vi "Initialization VI.vi"(8 "error in (no error)":errorcluster, 10 "Custom XML":string, 11 "Device Item Ref in":T1 format="%.0x") -> (0 "error out":errorcluster, 3 "Device Item Ref out":T1 format="%.0x")   [LabVIEW 2019, in "SLSC-12201 DIO System Explorer.lvlib"]
uses:
  SLSC-12201 DIO System Explorer.lvlib
  <vilib>/NI VeriStand/Custom Device API/Custom Device Item Ref.ctl
  Shared/Constants.vi
  <vilib>/NI VeriStand/Custom Device API/Set Item Property (String).vi
  <vilib>/NI VeriStand/Custom Device API/Set Item Property (U32).vi
  <vilib>/NI VeriStand/Custom Device API/Set Item Property (I32).vi
  <vilib>/NI VeriStand/Custom Device API/Get Item Property (Boolean).vi
  <vilib>/NI VeriStand/Custom Device API/Custom Device API.lvlib
  Shared/SLSC-12201 DIO Shared.lvlib
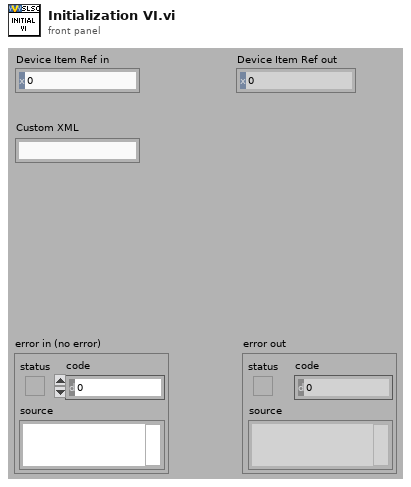
[diagram p1: front panel]
types:
  T1 = typedef "Custom Device API.lvlib/Custom Device Item Ref.ctl" = u64
  T2 = typedef "Custom Device API.lvlib/Custom Device Channel.ctl" = cluster{"Type":T3, "Units":string, "Default Value":dbl, "Faultable":bool, "Scalable":bool}
  T3 = typedef "Custom Device API.lvlib/Custom Device Channel Type.ctl" = enum16{"Input", "Output"}
  T4 = cluster{"Channel Name":string, "SLSC Name":string, "Channel":T2}[]
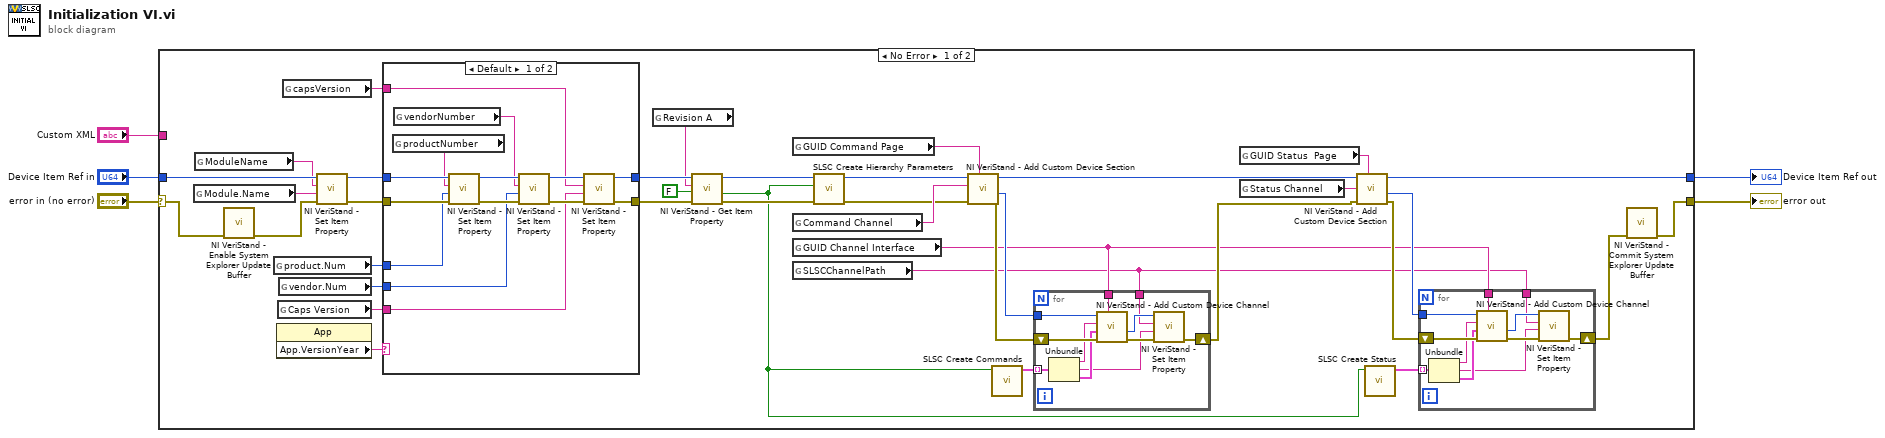
[diagram p0: block diagram]
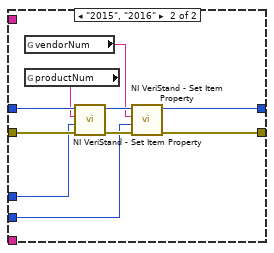
[diagram p2: hidden frame]
diagram:
  n1 = case shown="No Error" "error in (no error)" {
    selector: "error in (no error)" -> [w16 w91]
    tunnel: [w13 w91] -> w5
    tunnel: [w24 w90] -> w3
    tunnel: "Device Item Ref in" -> [w41 w90]
    tunnel: "Custom XML" -> [_ _]
    frame No Error {
      n2 = global read "Constants.vi" "Module.Name"() -> (w39:string)
      n3 = global read "Constants.vi" "ModuleName"() -> (w40:string)
      n4 = call <vilib>:"NI VeriStand - Enable System Explorer Update Buffer.vi"("error in (no error)"=w16) -> ("error out"=w15:errorcluster)  [unwired: 10 in]
      n5 = global read "Constants.vi" "product.Num"() -> (w38:i32)
      n6 = property class="App"() -> ("App.VersionYear"=w19:string)  [unwired: 2 in, 2 out]
      n7 = global read "Constants.vi" "Caps Version"() -> (w17:string)
      n8 = global read "Constants.vi" "vendor.Num"() -> (w37:i32)
      n9 = global read "Constants.vi" "capsVersion"() -> (w18:string)
      n10 = call-poly <vilib>:"NI VeriStand - Set Item Property.vi"("error in (no error)"=w15, "Value"=w39, "Property Name"=w40, "Item Ref in"=w41) -> ("error out"=w42:errorcluster, "Item Ref out"=w43:T1)  [unwired: 5 in, 1 out]
      n11 = case shown="Default" w19 {
        tunnel: w43 -> [w57 w67]
        tunnel: w42 -> [w55 w65]
        tunnel: [w50 w63] -> w12
        tunnel: [w48 w62] -> w11
        tunnel: w38 -> [w53 w61]
        tunnel: w37 -> [w52 w60]
        tunnel: w18 -> [w47 _]
        tunnel: w17 -> [w46 _]
        frame Default {
          n12 = global read "Constants.vi" "productNumber"() -> (w45:string)
          n13 = global read "Constants.vi" "vendorNumber"() -> (w44:string)
          n14 = call-poly <vilib>:"NI VeriStand - Set Item Property.vi"("error in (no error)"=w55, "Value"=w53, "Property Name"=w45, "Item Ref in"=w57) -> ("error out"=w54:errorcluster, "Item Ref out"=w56:T1)  [unwired: 5 in, 1 out]
          n15 = call-poly <vilib>:"NI VeriStand - Set Item Property.vi"("error in (no error)"=w54, "Value"=w52, "Property Name"=w44, "Item Ref in"=w56) -> ("error out"=w49:errorcluster, "Item Ref out"=w51:T1)  [unwired: 5 in, 1 out]
          n16 = call-poly <vilib>:"NI VeriStand - Set Item Property.vi"("error in (no error)"=w49, "Value"=w46, "Property Name"=w47, "Item Ref in"=w51) -> ("error out"=w48:errorcluster, "Item Ref out"=w50:T1)  [unwired: 5 in, 1 out]
        }
        frame "2015", "2016" {
          n17 = global read "Constants.vi" "vendorNum"() -> (w58:string)
          n18 = global read "Constants.vi" "productNum"() -> (w59:string)
          n19 = call-poly <vilib>:"NI VeriStand - Set Item Property.vi"("error in (no error)"=w65, "Value"=w61, "Property Name"=w59, "Item Ref in"=w67) -> ("error out"=w64:errorcluster, "Item Ref out"=w66:T1)  [unwired: 5 in, 1 out]
          n20 = call-poly <vilib>:"NI VeriStand - Set Item Property.vi"("error in (no error)"=w64, "Value"=w60, "Property Name"=w58, "Item Ref in"=w66) -> ("error out"=w62:errorcluster, "Item Ref out"=w63:T1)  [unwired: 5 in, 1 out]
        }
      }
      n21 = global read "Constants.vi" "Revision A"() -> (w7:string)
      n22 = call-poly <vilib>:"NI VeriStand - Get Item Property.vi"("error in (no error)"=w11, "Default Value"=FALSE, "Property Name"=w7, "Item Ref in"=w12) -> ("error out"=w8:errorcluster, "Value"=w6:bool, "Item Ref out"=w9:T1)  [unwired: 4 in, 1 out]
      n23 = global read "Constants.vi" "GUID Command Page"() -> (w30:string)
      n24 = global read "Constants.vi" "Command Channel"() -> (w29:string)
      n25 = global read "Constants.vi" "GUID Channel Interface"() -> (w21:string)
      n26 = global read "Constants.vi" "SLSCChannelPath"() -> (w20:string)
      n27 = call "SLSC Create Hierarchy Parameters.vi"("error in (no error)"=w8, "RevA?"=w6, "Item Ref in"=w9) -> ("error out"=w22:errorcluster, "Item Ref out"=w23:T1)  [unwired: 7 in]
      n28 = call <vilib>:"NI VeriStand - Add Custom Device Section.vi"("GUID (Default Section)"=w30, "error in (no error)"=w22, "Section Name"=w29, "Parent Ref in"=w23) -> ("error out"=w31:errorcluster, "Section Ptr"=w32:T1, "Parent Ref out"=w25:T1)  [unwired: 4 in, 1 out]
      n29 = call "SLSC Create Commands.vi"("RevA?"=w6) -> ("Outgoing configuration"=w28:T4)  [unwired: 10 in]
      n30 = for {
        tunnel: w32 -> [w73]
        shift-right: [w76] -> w26
        shift-left: w31 -> [w72]
        tunnel: w20 -> [w75]
        tunnel: w21 -> [w74]
        tunnel: w28 -> [w71] mode=indexing
        n31 = Unbundle(w71) -> ("Channel Name"=w70:string, "SLSC Name"=w68:string, "Channel"=w69:T2)
        n32 = call <vilib>:"NI VeriStand - Add Custom Device Channel.vi"("GUID (Default Channel)"=w74, "error in (no error)"=w72, "Channel"=w69, "Channel Name"=w70, "Parent Ref in"=w73) -> ("error out"=w77:errorcluster, "Channel Ref"=w78:T1)  [unwired: 3 in, 2 out]
        n33 = call-poly <vilib>:"NI VeriStand - Set Item Property.vi"("error in (no error)"=w77, "Value"=w68, "Property Name"=w75, "Item Ref in"=w78) -> ("error out"=w76:errorcluster)  [unwired: 5 in, 2 out]
      }
      n34 = global read "Constants.vi" "GUID Status  Page"() -> (w33:string)
      n35 = global read "Constants.vi" "Status Channel"() -> (w36:string)
      n36 = call <vilib>:"NI VeriStand - Add Custom Device Section.vi"("GUID (Default Section)"=w33, "error in (no error)"=w26, "Section Name"=w36, "Parent Ref in"=w25) -> ("error out"=w35:errorcluster, "Section Ptr"=w34:T1, "Parent Ref out"=w24:T1)  [unwired: 4 in, 1 out]
      n37 = call "SLSC Create Status.vi"("RevA?"=w6) -> ("Outgoing configuration"=w27:T4)  [unwired: 10 in]
      n38 = for {
        tunnel: w34 -> [w84]
        shift-right: [w87] -> w14
        shift-left: w35 -> [w83]
        tunnel: w20 -> [w86]
        tunnel: w21 -> [w85]
        tunnel: w27 -> [w82] mode=indexing
        n39 = Unbundle(w82) -> ("Channel Name"=w81:string, "SLSC Name"=w79:string, "Channel"=w80:T2)
        n40 = call <vilib>:"NI VeriStand - Add Custom Device Channel.vi"("GUID (Default Channel)"=w85, "error in (no error)"=w83, "Channel"=w80, "Channel Name"=w81, "Parent Ref in"=w84) -> ("error out"=w88:errorcluster, "Channel Ref"=w89:T1)  [unwired: 3 in, 2 out]
        n41 = call-poly <vilib>:"NI VeriStand - Set Item Property.vi"("error in (no error)"=w88, "Value"=w79, "Property Name"=w86, "Item Ref in"=w89) -> ("error out"=w87:errorcluster)  [unwired: 5 in, 2 out]
      }
      n42 = call <vilib>:"NI VeriStand - Commit System Explorer Update Buffer.vi"("error in (no error)"=w14) -> ("error out"=w13:errorcluster)  [unwired: 10 in]
    }
    frame Error {
    }
  }
  "error out" <- w5
  "Device Item Ref out" <- w3
